vi "Command Create.vi"   [LabVIEW 2017, in "Roboteq Controller KBL1xxx.lvlib"]
uses:
  <instrlib>/Roboteq Controller KBL1xxx/Roboteq Controller KBL1xxx.lvlib
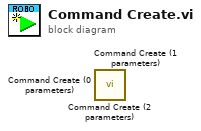
[diagram p0: block diagram]
diagram:
  n1 = call <instrlib>:"Command Create (2 parameters).vi"() -> ()  [unwired: 11 in, 1 out]
  n2 = call <instrlib>:"Command Create (1 parameters).vi"() -> ()  [unwired: 11 in, 1 out]
  n3 = call <instrlib>:"Command Create (0 parameters).vi"() -> ()  [unwired: 11 in, 1 out]
